vi "load.vi"(7 "progress bar ref":refnum<vi>, 8 "error in (no error)":errorcluster, 9 "Image Type":T1=4 items=["Grayscale (U8)", "Grayscale (I16)", "Grayscale (SGL)", "Complex (CSG)", "RGB (U32)", "HSL (U32)", "RGB (U64)", "Grayscale (U16)"], 10 "path in":path, 11 "ImageCollection in":refnum<class "ImageCollection.lvclass">) -> (0 "error out":errorcluster, 1 "path out":path, 2 "description":string, 3 "ImageCollection out":refnum<class "ImageCollection.lvclass">, 4 "description empty?":bool)   [LabVIEW 2010, in "ImageCollection.lvclass"]
uses:
  ImageCollection.lvclass
  XMLElement/XMLElement/XMLElement.lvclass
  ImageCollection.lvclass/ImageCollection.ctl
  type_enum.ctl
  add_mode_enum.ctl
  Image/Image/Image.lvclass
  libraries/TIFFManagement/TIFFManagement.lvlib
panel:
  out "cancelled?":bool
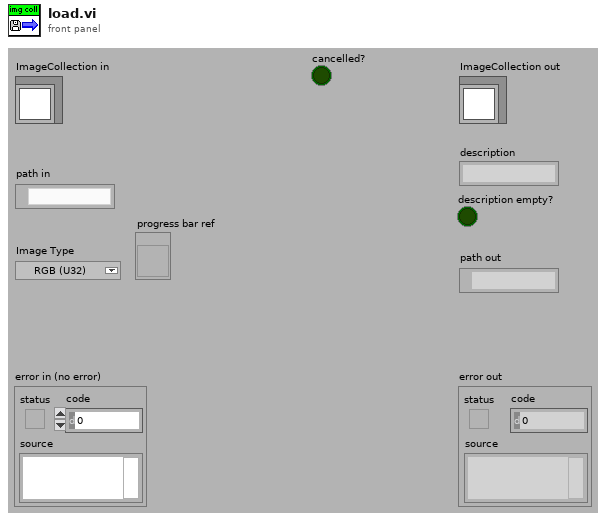
[diagram p1: front panel]
types:
  T1 = typedef "Image Type" = u32
  T2 = typedef "type_enum.ctl" = enum16{"undefined", "movie", "z-stack"}
  T3 = typedef "ImageCollection.lvclass/add_mode_enum.ctl" = enum16{"instance", "copy"}
  T4 = typedef "ImageCollection.lvclass/storage_mode_enum.ctl" = enum16{"RAM", "single files", "multipage TIFF (read-only)"}
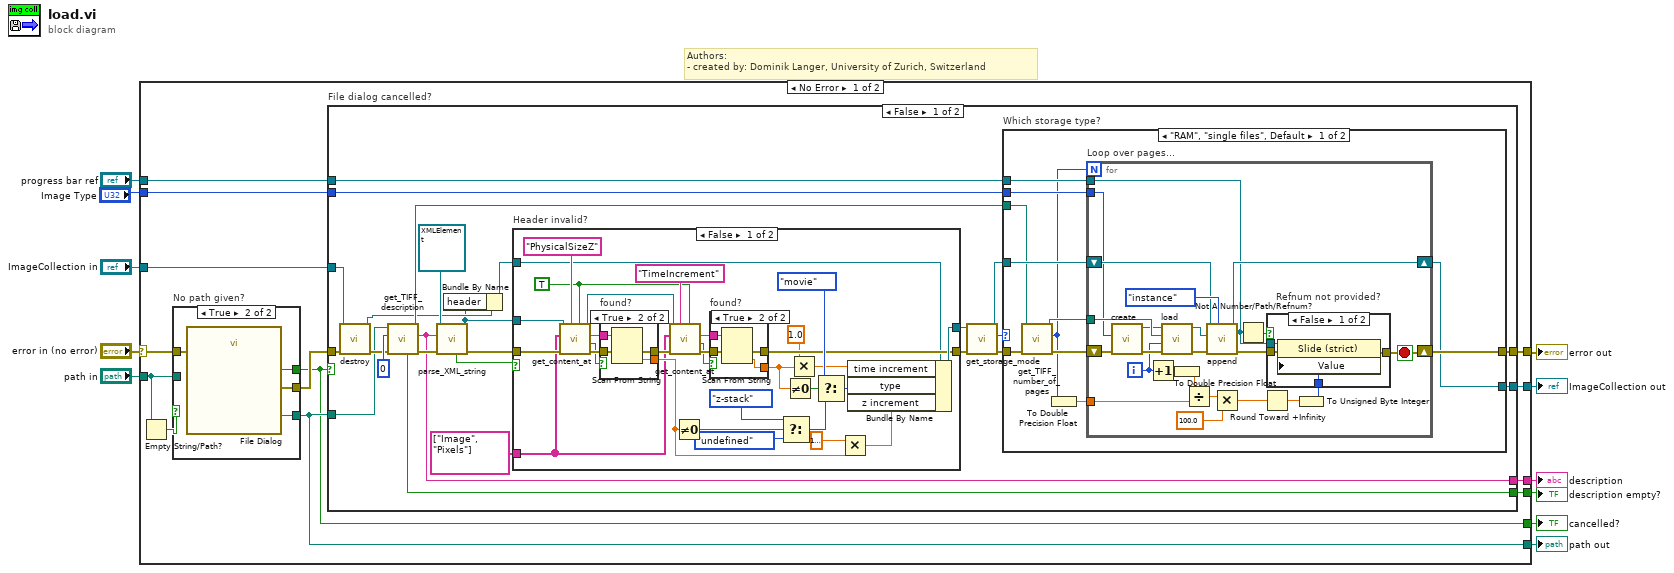
[diagram p0: block diagram]
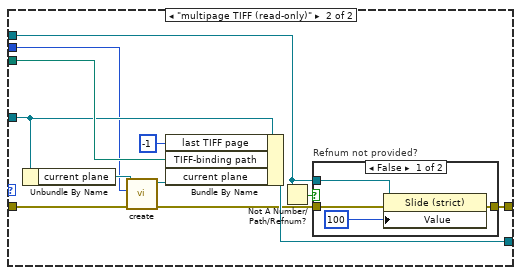
[diagram p6: hidden frame]
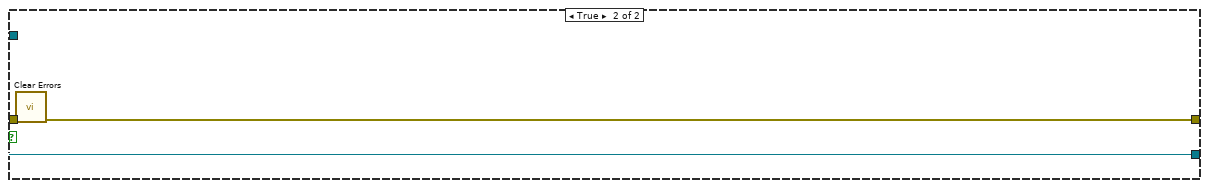
[diagram p8: hidden frame]
diagram:
  # "Authors: \n- created by: Dominik Langer, University of Zurich, Switzerland"
  n1 = case shown="No Error" "error in (no error)" {
    selector: "error in (no error)" -> [w23 w158]
    tunnel: [w17 w158] -> w10
    tunnel: [w18 w157] -> w8
    tunnel: "ImageCollection in" -> [w24 w157]
    tunnel: "path in" -> [w20 _]
    tunnel: [w16 _] -> w6
    tunnel: [w19 _] -> w5
    tunnel: [w15 _] -> w4
    tunnel: "Image Type" -> [w14 _]
    tunnel: [w13 _] -> w2
    tunnel: "progress bar ref" -> [w12 _]
    frame No Error {
      n2 = Empty String/Path?(string/path=w20) -> (empty?=w21:bool)
      n3 = case "No path given?" shown="True" w21 {
        tunnel: w23 -> [w151 w156]
        tunnel: [w151 w155] -> w22
        tunnel: [w152 w154] -> w15
        tunnel: w20 -> [w152 _]
        tunnel: [_ w153] -> w13
        frame False {
        }
        frame True {
          n4 = call "File Dialog"("error in"=w156) -> ("selected path"=w154:path, "cancelled"=w153:bool, "error out"=w155:errorcluster)  [unwired: 11 in, 1 out]
        }
      }
      n5 = case "File dialog cancelled?" shown="False" w13 {
        tunnel: w24 -> [w40 w150]
        tunnel: w22 -> [w41 w149]
        tunnel: [w39 _] -> w19
        tunnel: [w49 w150] -> w18
        tunnel: [w48 w148] -> w17
        tunnel: [w28 _] -> w16
        tunnel: w15 -> [w38 _]
        tunnel: w14 -> [w47 _]
        tunnel: w12 -> [w36 _]
        frame False {
          n6 = call-dynamic "destroy.vi"("error in (no error)"=w41, "ImageCollection in"=w40) -> ("error out"=w42:errorcluster, "ImageCollection out"=w33:refnum<class "ImageCollection.lvclass">)  [unwired: 8 in]
          n7 = call "get_TIFF_description.vi"("error in (no error)"=w42, "page"=0, "path in"=w38) -> ("error out"=w34:errorcluster, "description"=w28:string, "path out"=w37:path, "description empty?"=w39:bool)  [unwired: 5 in]
          n8 = call "parse_XML_string.vi"("error in (no error)"=w34, "XML string"=w28, "Element in"=refnum<class "XMLElement.lvclass"> refnum ("XMLElement.lvclass")) -> ("error out"=w32:errorcluster, "Element out"=w27:refnum<class "XMLElement.lvclass">, "header empty or invalid XML?"=w25:bool)  [unwired: 6 in]
          n9 = Bundle By Name(cluster=w33, "header"=w27) -> (w30:refnum<class "ImageCollection.lvclass">)
          n10 = case "Header invalid?" shown="False" w25 {
            tunnel: [w76 w91] -> w29
            tunnel: string[] ["Image", "Pixels"] ("key chain") -> [w50 _]
            tunnel: [w63 w90] -> w31
            tunnel: w32 -> [w53 w90]
            tunnel: w30 -> [w52 w91]
            tunnel: w27 -> [w51 _]
            frame False {
              w75 = TRUE ("ignore IDs")
              n11 = call "get_content_at.vi"("ignore IDs"=w75, "attribute name"="PhysicalSizeZ", "error in (no error)"=w53, "key chain"=w50, "Element in"=w51) -> ("error out"=w74:errorcluster, "found?"=w71:bool, "string"=w72:string, "Element out"=w77:refnum<class "XMLElement.lvclass">)  [unwired: 3 in]
              n12 = case "found?" shown="True" w71 {
                tunnel: w74 -> [w85 w89]
                tunnel: [w85 w88] -> w73
                tunnel: w72 -> [_ w87]
                tunnel: [_ w86] -> w60
                frame False {
                }
                frame True {
                  n13 = Scan From String(input string=w87, error in=w89) -> (error out=w88:errorcluster, output 1=w86:dbl)  [unwired: 3 in, 2 out]
                }
              }
              n14 = call "get_content_at.vi"("ignore IDs"=w75, "attribute name"="TimeIncrement", "error in (no error)"=w73, "key chain"=w50, "Element in"=w77) -> ("error out"=w70:errorcluster, "found?"=w69:bool, "string"=w68:string)  [unwired: 3 in, 1 out]
              n15 = Not Equal To 0?(x=w60) -> (x != 0?=w67:bool)
              n16 = case "found?" shown="True" w69 {
                tunnel: w70 -> [w80 w84]
                tunnel: [w80 w83] -> w63
                tunnel: w68 -> [_ w82]
                tunnel: [_ w81] -> w54
                frame False {
                }
                frame True {
                  n17 = Scan From String(input string=w82, error in=w84) -> (error out=w83:errorcluster, output 1=w81:dbl)  [unwired: 3 in, 2 out]
                }
              }
              n18 = Select(t=type_enum."z-stack" ("type"), s=w67, f=type_enum."undefined" ("type")) -> (s? t:f=w64:T2)
              n19 = Not Equal To 0?(x=w54) -> (x != 0?=w66:bool)
              n20 = Multiply(x=dbl[unit] 1.0 ("unit (none)"), y=w54) -> (x*y=w57:dbl[unit])
              n21 = Select(t=type_enum."movie" ("type"), s=w66, f=w64) -> (s? t:f=w55:T2)
              n22 = Multiply(x=dbl[unit] 1e-06, y=w60) -> (x*y=w58:dbl[unit])
              n23 = Bundle By Name(cluster=w52, "time increment"=w57, "type"=w55, "z increment"=w58) -> (w76:refnum<class "ImageCollection.lvclass">)
            }
            frame True {
            }
          }
          n24 = call-dynamic "get_storage_mode.vi"("error in (no error)"=w31, "ImageCollection.lvclass in"=w29) -> ("error out"=w46:errorcluster, "storage type"=w44:T4, "ImageCollection.lvclass out"=w45:refnum<class "ImageCollection.lvclass">)  [unwired: 7 in]
          n25 = case "Which storage type?" shown="\"RAM\", \"single files\", Default" w44 {
            tunnel: [w92 w141] -> w49
            tunnel: [w93 w133] -> w48
            tunnel: w37 -> [w97 w142]
            tunnel: w47 -> [w100 w136]
            tunnel: w46 -> [w98 w139]
            tunnel: w45 -> [w99 w140]
            tunnel: w36 -> [w96 w131]
            frame "RAM", "single files", Default {
              n26 = call "get_TIFF_number_of_pages.vi"("error in (no error)"=w98, "path in"=w97) -> ("error out"=w102:errorcluster, "number of pages"=w95:i32, "path out"=w101:path)  [unwired: 7 in]
              n27 = To Double Precision Float(number=w95) -> (double precision float=w94:dbl)
              n28 = for "Loop over pages..." {
                N: w95 -> [_]
                shift-right: [w103] -> w93
                shift-left: w102 -> [w119]
                tunnel: w101 -> [w125]
                shift-right: [w122] -> w92
                shift-left: w99 -> [w121]
                tunnel: w100 -> [w116]
                tunnel: w96 -> [w107]
                tunnel: w94 -> [w113]
                i -> [w105]
                stop <- w103 stop-if-true
                n29 = call "create.vi"("error in (no error)"=w119, "Image Type"=w116) -> ("error out"=w118:errorcluster, "Image out"=w117:refnum<class "Image.lvclass">)  [unwired: 8 in]
                n30 = Increment(x=w105) -> (x+1=w104:i32)
                n31 = call-dynamic "load.vi"("error in (no error)"=w118, "page"=w105, "Path"=w125, "Image in"=w117) -> ("error out"=w124:errorcluster, "Image out"=w120:refnum<class "Image.lvclass">)  [unwired: 4 in, 2 out]
                n32 = To Double Precision Float(number=w104) -> (double precision float=w114:dbl)
                n33 = Divide(x=w114, y=w113) -> (x/y=w112:dbl)
                n34 = call-dynamic "append.vi"("add mode"=add_mode_enum."instance", "error in (no error)"=w124, "Image.lvclass"=w120, "ImageCollection in"=w121) -> ("error out"=w115:errorcluster, "ImageCollection out"=w122:refnum<class "ImageCollection.lvclass">)  [unwired: 5 in, 1 out]
                n35 = Multiply(x=w112, y=100.0) -> (x*y=w111:dbl)
                n36 = Not A Number/Path/Refnum?(number/path/refnum=w107) -> (NaN/Path/Refnum?=w106:bool)
                n37 = Round Toward +Infinity(x=w111) -> (ceil(x): smallest int >= x=w110:dbl)
                n38 = To Unsigned Byte Integer(number=w110) -> (unsigned 8bit integer=w109:u8)
                n39 = case "Refnum not provided?" shown="False" w106 {
                  tunnel: w107 -> [w129 _]
                  tunnel: w115 -> [w128 w130]
                  tunnel: [w127 w130] -> w103
                  tunnel: w109 -> [w126 _]
                  frame False {
                    n40 = property class="Slide (strict)"(reference=w129, error in=w128, "Value"=w126) -> (error out=w127:errorcluster)  [unwired: 1 out]
                  }
                  frame True {
                  }
                }
              }
            }
            frame "multipage TIFF (read-only)" {
              n41 = Unbundle By Name(w140) -> ("current plane"=w137:refnum<class "Image.lvclass">)
              n42 = call "create.vi"("error in (no error)"=w139, "Image Type"=w136, "Image in"=w137) -> ("error out"=w134:errorcluster, "Image out"=w138:refnum<class "Image.lvclass">)  [unwired: 7 in]
              n43 = Bundle By Name(cluster=w140, "last TIFF page"=-1 ("current image index"), "TIFF-binding path"=w142, "current plane"=w138) -> (w141:refnum<class "ImageCollection.lvclass">)
              n44 = Not A Number/Path/Refnum?(number/path/refnum=w131) -> (NaN/Path/Refnum?=w132:bool)
              n45 = case "Refnum not provided?" shown="False" w132 {
                tunnel: w134 -> [w146 w147]
                tunnel: [w145 w147] -> w133
                tunnel: w131 -> [w143 _]
                frame False {
                  n46 = property class="Slide (strict)"(reference=w143, error in=w146, "Value"=u8 100) -> (error out=w145:errorcluster)  [unwired: 1 out]
                }
                frame True {
                }
              }
            }
          }
        }
        frame True {
          n47 = call <vilib>:"Clear Errors.vi"("error in (no error)"=w149) -> ("error out"=w148:errorcluster)  [unwired: 6 in]
        }
      }
    }
    frame Error {
    }
  }
  "error out" <- w10
  "ImageCollection out" <- w8
  "description" <- w6
  "description empty?" <- w5
  "path out" <- w4
  "cancelled?" <- w2
